vi "add_data_path_system.vi"(8 "error in (no error)":errorcluster, 11 "relative_path_file":path) -> (0 "error out":errorcluster)   [LabVIEW 2015, in "lv-bin.lvlib" / "v1.lvlib"]
uses:
  v1.lvlib
  private/_controls/fg_command.ctl
  lv-bin.lvlib
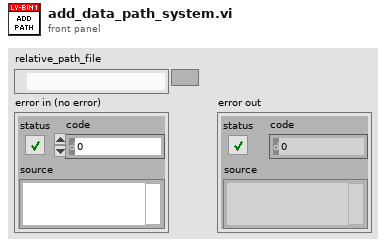
[diagram p1: front panel]
types:
  T1 = typedef "lv-bin.lvlib/fg_command.ctl" = enum16{"<fg_command>", "initialize", "read", "write", "shutdown", "<null>"}
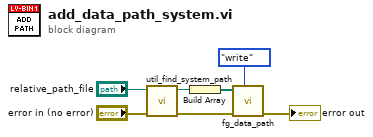
[diagram p0: block diagram]
diagram:
  n1 = call "util_find_system_path.vi"("error in (no error)"="error in (no error)", "relative_path_file"="relative_path_file") -> ("error out"=w3:errorcluster, "system_path"=w2:path)  [unwired: 6 in, 2 out]
  n2 = Build Array(w2) -> (w5:path[])
  n3 = call "fg_data_path.vi"("fg_command"=fg_command."write", "error in (no error)"=w3, "path [] in"=w5) -> ("error out"=→"error out":errorcluster)  [unwired: 7 in, 1 out]
